vi "ButtonState2Color.vi"(11 "ButtonState":u8) -> (3 "Color":u32)   [LabVIEW 2020]
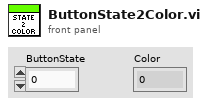
[diagram p1: front panel]
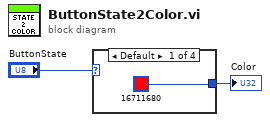
[diagram p0: block diagram]
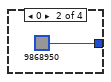
[diagram p2: hidden frame]
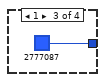
[diagram p3: hidden frame]
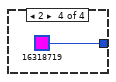
[diagram p4: hidden frame]
diagram:
  n1 = case shown="Default" "ButtonState" {
    tunnel: [u32 16711680 u32 9868950 u32 2777087 u32 16318719] -> w2
    frame Default {
    }
    frame 0 {
    }
    frame 1 {
    }
    frame 2 {
    }
  }
  "Color" <- w2
